vi "rad_ReadTargetConfigOptions.vi"(8 "error in (no error)":errorcluster, 11 "configuration file path":path) -> (0 "error out":errorcluster, 3 "TargetConfigurationOptions":T1={"NumInBatch"=0, "Target Config Operation"=enum."No Config", "Target Name"="", "Increment Static IPs"=FALSE, "Change Target Name"=FALSE, "Primary NIC"={"MAC address"="", "IP Address Request Mode"=2, "IP address"="", "Subnet mask"="", "Gateway"="", "DNS server"=""}} {"Primary NIC"."IP Address Request Mode" items=["Static"=1, "DHCP/Link-Local"=2, "Link-Local Only"=4, "DHCP Only"=8]})   [LabVIEW 2013]
uses:
  App Images/TypeDefs/rad_Target Configuration Settings.ctl
  App Images/TypeDefs/rad_Target Configuration Operations.ctl
  TypeDefs/rad_Target Network Settings.ctl
  <vilib>/Utility/config.llb/Read Key (U32).vi
  <vilib>/Utility/config.llb/Read Key (String).vi
  <vilib>/Utility/config.llb/Read Key (Boolean).vi
  <vilib>/Utility/config.llb/Read Key (I32).vi
  <vilib>/Utility/config.llb/NI_LVConfig.lvlib
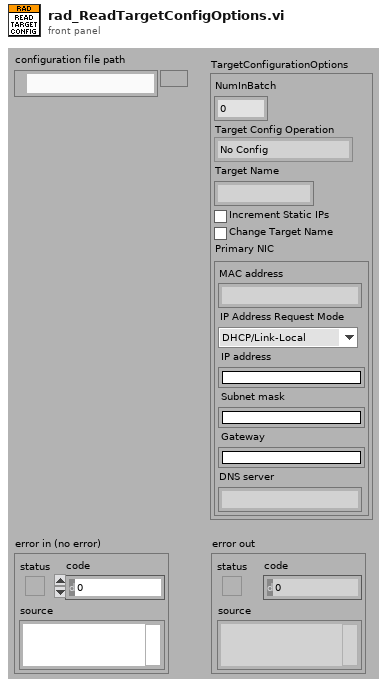
[diagram p1: front panel]
types:
  T1 = typedef "rad_Target Configuration Settings.ctl" = cluster{"NumInBatch":u32, "Target Config Operation":T2, "Target Name":string, "Increment Static IPs":bool, "Change Target Name":bool, "Primary NIC":T3}
  T2 = typedef "rad_Target Configuration Operations.ctl" = enum8{"No Config", "Image Config", "Static Config"}
  T3 = typedef "rad_Target Network Settings.ctl" = cluster{"MAC address":string, "IP Address Request Mode":i32, "IP address":string, "Subnet mask":string, "Gateway":string, "DNS server":string}
  T4 = typedef "NI_LVConfig.lvlib/Config Data RefNum.ctl" = refnum<k1>
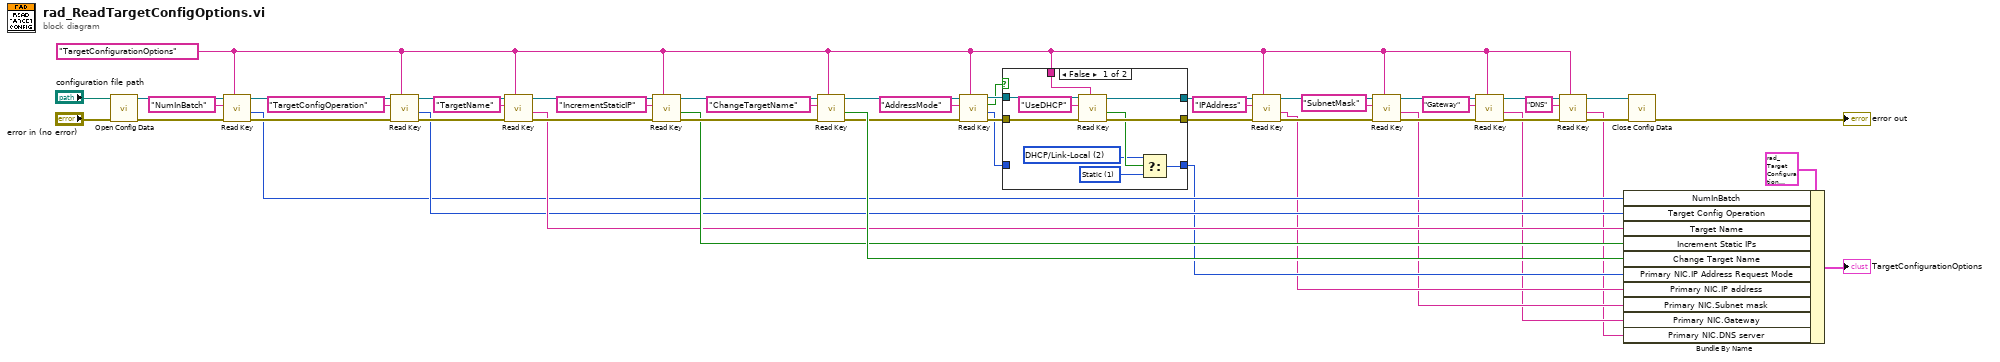
[diagram p0: block diagram]
diagram:
  w1 = "TargetConfigurationOptions" ("section")
  n1 = call <vilib>:"Open Config Data.vi"("error in (no error)"="error in (no error)", "configuration file path"="configuration file path") -> ("error out"=w50:errorcluster, "refnum"=w51:T4)  [unwired: 7 in, 1 out]
  n2 = call-poly <vilib>:"Read Key.vi"("section"=w1, "error in (no error)"=w50, "key"="NumInBatch", "refnum"=w51) -> ("error out"=w46:errorcluster, "value"=w21:u32, "refnum out"=w47:T4)  [unwired: 4 in, 1 out]
  n3 = call-poly <vilib>:"Read Key.vi"("section"=w1, "error in (no error)"=w46, "key"="TargetConfigOperation", "refnum"=w47) -> ("error out"=w44:errorcluster, "value"=w22:u32, "refnum out"=w43:T4)  [unwired: 4 in, 1 out]
  n4 = call-poly <vilib>:"Read Key.vi"("section"=w1, "error in (no error)"=w44, "key"="TargetName", "refnum"=w43) -> ("error out"=w32:errorcluster, "value"=w23:string, "refnum out"=w19:T4)  [unwired: 4 in, 1 out]
  n5 = call-poly <vilib>:"Read Key.vi"("section"=w1, "error in (no error)"=w32, "key"="IncrementStaticIP", "refnum"=w19) -> ("error out"=w31:errorcluster, "value"=w24:bool, "refnum out"=w18:T4)  [unwired: 4 in, 1 out]
  n6 = call-poly <vilib>:"Read Key.vi"("section"=w1, "error in (no error)"=w31, "key"="ChangeTargetName", "refnum"=w18) -> ("error out"=w13:errorcluster, "value"=w25:bool, "refnum out"=w12:T4)  [unwired: 4 in, 1 out]
  n7 = call-poly <vilib>:"Read Key.vi"("section"=w1, "error in (no error)"=w13, "key"="AddressMode", "refnum"=w12) -> ("error out"=w10:errorcluster, "value"=w7:i32, "found?"=w8:bool, "refnum out"=w11:T4)  [unwired: 4 in]
  n8 = case shown="False" w8 {
    tunnel: [w61 w63] -> w30
    tunnel: w1 -> [w60 _]
    tunnel: [w59 w64] -> w17
    tunnel: w11 -> [w58 w64]
    tunnel: w10 -> [w57 w63]
    tunnel: w7 -> [_ w65]
    tunnel: [w56 w65] -> w6
    frame False {
      w53 = 1 items=["Static"=1, "DHCP/Link-Local"=2, "Link-Local Only"=4, "DHCP Only"=8] ("IP Address Request Mode")
      w54 = 2 items=["Static"=1, "DHCP/Link-Local"=2, "Link-Local Only"=4, "DHCP Only"=8] ("IP Address Request Mode")
      n9 = call-poly <vilib>:"Read Key.vi"("section"=w60, "error in (no error)"=w57, "key"="UseDHCP", "refnum"=w58) -> ("error out"=w61:errorcluster, "value"=w55:bool, "refnum out"=w59:T4)  [unwired: 4 in, 1 out]
      n10 = Select(t=w54, s=w55, f=w53) -> (s? t:f=w56:i32)
    }
    frame True {
    }
  }
  n11 = call-poly <vilib>:"Read Key.vi"("section"=w1, "error in (no error)"=w30, "key"="IPAddress", "refnum"=w17) -> ("error out"=w28:errorcluster, "value"=w5:string, "refnum out"=w16:T4)  [unwired: 4 in, 1 out]
  n12 = call-poly <vilib>:"Read Key.vi"("section"=w1, "error in (no error)"=w28, "key"="SubnetMask", "refnum"=w16) -> ("error out"=w27:errorcluster, "value"=w4:string, "refnum out"=w15:T4)  [unwired: 4 in, 1 out]
  n13 = call-poly <vilib>:"Read Key.vi"("section"=w1, "error in (no error)"=w27, "key"="Gateway", "refnum"=w15) -> ("error out"=w26:errorcluster, "value"=w3:string, "refnum out"=w14:T4)  [unwired: 4 in, 1 out]
  n14 = call-poly <vilib>:"Read Key.vi"("section"=w1, "error in (no error)"=w26, "key"="DNS", "refnum"=w14) -> ("error out"=w36:errorcluster, "value"=w2:string, "refnum out"=w35:T4)  [unwired: 4 in, 1 out]
  n15 = Bundle By Name(cluster=T1 {"NumInBatch"=0, "Target Config Operation"=enum."No Config", "Target Name"="", "Increment Static IPs"=FALSE, "Change Target Name"=FALSE, "Primary NIC"={"MAC address"="", "IP Address Request Mode"=0, "IP address"="", "Subnet mask"="", "Gateway"="", "DNS server"=""}} ("Target Configuration Options"), "NumInBatch"=w21, "Target Config Operation"=w22, "Target Name"=w23, "Increment Static IPs"=w24, "Change Target Name"=w25, "Primary NIC.IP Address Request Mode"=w6, "Primary NIC.IP address"=w5, "Primary NIC.Subnet mask"=w4, "Primary NIC.Gateway"=w3, "Primary NIC.DNS server"=w2) -> (→"TargetConfigurationOptions":T1)
  n16 = call <vilib>:"Close Config Data.vi"("error in (no error)"=w36, "refnum"=w35) -> ("error out"=→"error out":errorcluster)  [unwired: 8 in, 1 out]
